vi "CSM - Get New State Notifier Event.vi"(8 "Error in":errorcluster caption="Error in (no error)", 11 "Name(\"\" to use uuid) in":string) -> (0 "Error out":errorcluster, 3 "New State Notifier Event":refnum<user-event>)   [LabVIEW 2020, in "Communicable State Machine.lvlib"]
doc: "<b>Inputs:</b>\n - <b>Name(\"\" to use uuid) in</b>: CSM module name\n - <b>Error in</b>: Error cluster\n\n<b>Outputs:</b>\n - <b>New State Notifier Event</b>: User event to break CSM module from waiting in event structure when message is received.\n - <b>Error out</b>: Error cluster"
uses:
  Communicable State Machine.lvlib
  _CSMOFGVOPER.ctl
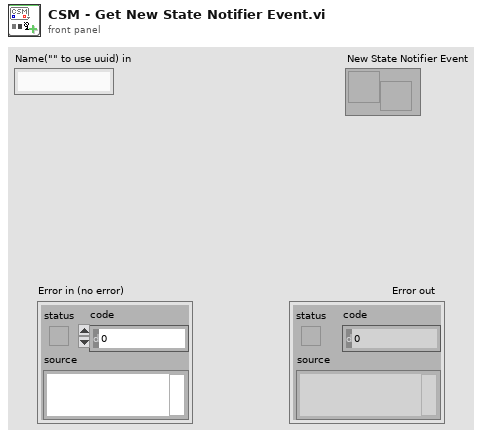
[diagram p1: front panel]
types:
  T1 = typedef "Communicable State Machine.lvlib/_CSMOFGVOPER.ctl" = enum16{"Create If not Exist", "Get By Name", "List", "Check If Name Exists", "Release", "Module Status", "Create Status Event Handler", "Destroy Status Event Handler"}
  T2 = typedef "Communicable State Machine.lvlib/_CSMObj.ctl" = cluster{"Requested Name":string, "Module Name":string, "Mode":T3, "Queue":refnum<class "Priority Queue.lvclass">, "CSM-Data":refnum<data-value>, "User Event":refnum<user-event>, "Status Change Event":refnum<user-event>, "Allowed Messages":string[], "Mode-Data":refnum<data-value>, "Group Name":string, "Exit Event":refnum<user-event>}
  T3 = typedef "Communicable State Machine.lvlib/_CSM_MODE.ctl" = enum16{"Not Exist", "Stand Alone", "CSM", "Worker Agent", "Worker", "Chain", "Chain Node"}
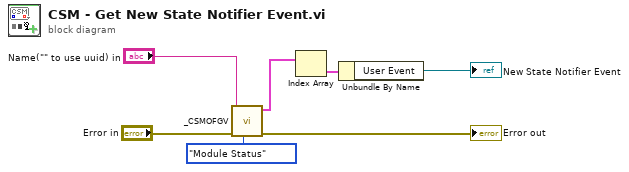
[diagram p0: block diagram]
diagram:
  n1 = call "_CSMOFGV.vi"("Operation"=_CSMOFGVOPER."Module Status", "Error in"="Error in", "Name(\"\" to use uuid) in"="Name(\"\" to use uuid) in") -> ("Error out"=→"Error out":errorcluster, "Array"=w3:T2[])  [unwired: 6 in, 1 out]
  n2 = Index Array(array=w3) -> (element=w2:T2)  [unwired: 1 in]
  n3 = Unbundle By Name(w2) -> ("User Event"=→"New State Notifier Event":refnum<user-event>)
